vi "file -- read list of lines.vi"(8 "file name":string, 11 "folder path":path) -> (1 "text lines":string[](array[string]))   [LabVIEW 2015]
uses:
  <vilib>/Utility/file.llb/Read From Spreadsheet File (string).vi
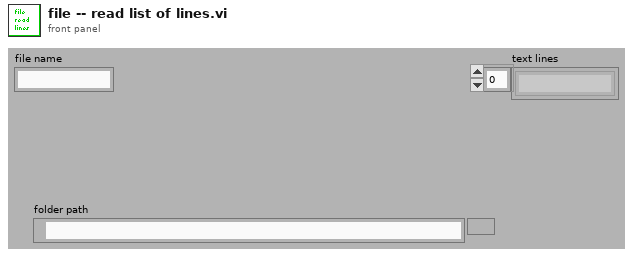
[diagram p1: front panel]
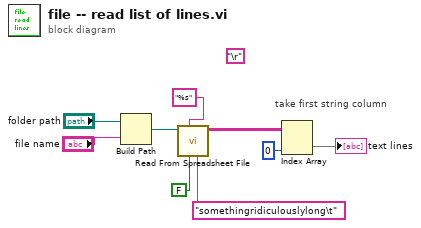
[diagram p0: block diagram]
diagram:
  (unwired) "\r"
  # "take first string column"
  n1 = Build Path(base path="folder path", name or relative path="file name") -> (appended path=w4:path)
  n2 = call-poly <vilib>:"Read From Spreadsheet File.vi"("delimiter (\\t)"="somethingridiculouslylong\t" ("delimiter (\\t)"), "transpose (no:F)"=FALSE ("append to file? (new file:F)"), "format (%s)"="%s", "file path (dialog if empty)"=w4) -> ("all rows"=w6:string[][])  [unwired: 3 in, 4 out]
  n3 = Index Array(array=w6, index (col)=0 ("disabled index (col)")) -> (element=→"text lines":string[])  [unwired: 1 in]
